vi "Vitrek Enable Interlock.vi"(8 "error in (no error)":errorcluster, 11 "VISA resource name in":refnum<visa-resource-name>="COM13") -> (0 "error out":errorcluster)   [LabVIEW 2018]
uses:
  <vilib>/Instr/_visa.llb/VISA Configure Serial Port (Instr).vi
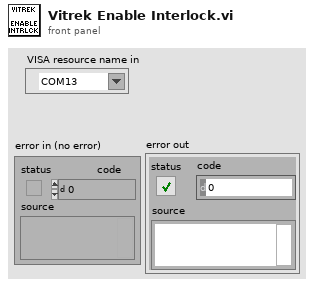
[diagram p1: front panel]
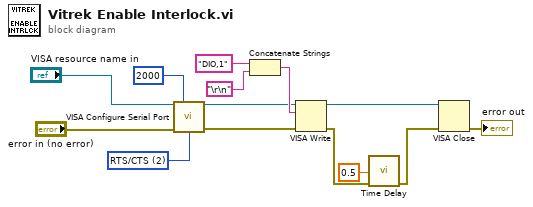
[diagram p0: block diagram]
diagram:
  w13 = u16 2 items=["None", "XON/XOFF", "RTS/CTS", "XON/XOFF & RTS/CTS", "DTR/DSR", "XON/XOFF & DTR/DSR"] ("flow control (0:none)")
  n1 = call-poly "VISA Configure Serial Port"("VISA resource name"="VISA resource name in", "timeout (10sec)"=u32 2000, "error in (no error)"="error in (no error)", "flow control (0:none)"=w13) -> ("VISA resource name out"=w8:refnum<visa-resource-name>, "error out"=w9:errorcluster)  [unwired: 10 in]
  n2 = Concatenate Strings("DIO,1" ("write buffer"), "\r\n") -> (w10:string)
  n3 = VISA Write(VISA resource name=w8, write buffer=w10, error in (no error)=w9) -> (VISA resource name out=w2:refnum<visa-resource-name>, error out=w5:errorcluster)  [unwired: 1 out]
  n4 = call "Time Delay"("error in (no error)"=w5, "Delay Time (s)"=0.5) -> ("error out"=w3:errorcluster)  [unwired: 9 in]
  n5 = VISA Close(VISA resource name=w2, error in (no error)=w3) -> (error out=→"error out":errorcluster)
